vi "Core.vi"(8 "error in (no error)":errorcluster, 11 "Template in":refnum<class "Template.lvclass">) -> (0 "error out":errorcluster, 3 "Actor out":refnum<class "Actor.lvclass">)   [LabVIEW 2020, in "Artifex Template.lvlib" / "Template.lvclass"]
uses:
  Template.lvclass
  Artifex/Actor/Actor.lvclass
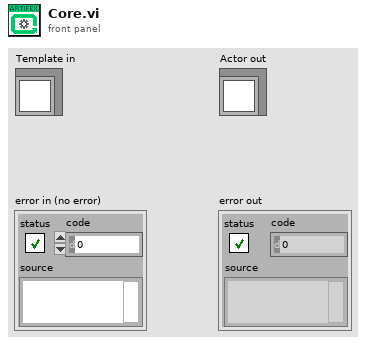
[diagram p1: front panel]
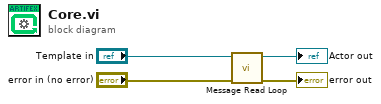
[diagram p0: block diagram]
diagram:
  n1 = call "Message Read Loop.vi"("error in (no error)"="error in (no error)", "Actor in"="Template in") -> ("error out"=→"error out":errorcluster, "Actor out"=→"Actor out":refnum<class "Actor.lvclass">)  [unwired: 8 in]
